vi "update_MagFieldTable_File.vi"(8 "error in (no error)":errorcluster, 11 "MFTObj in":refnum<class "MagFieldTable.lvclass">) -> (0 "error out":errorcluster, 3 "MFTObj out":refnum<class "MagFieldTable.lvclass">)   [LabVIEW 2018]
doc: "updates the MagFieldTables.ini with the most recent data of this MagFieldTable"
uses:
  Classes/MagFieldTable/MagFieldTable.lvclass
  global variables.vi
  <vilib>/Utility/config.llb/Write Key (Double).vi
  Classes/StatusLog/StatusLog.lvclass
  <vilib>/Utility/config.llb/NI_LVConfig.lvlib
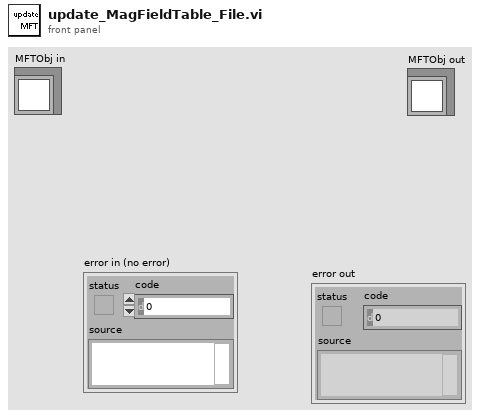
[diagram p1: front panel]
types:
  T1 = typedef "NI_LVConfig.lvlib/Config Data RefNum.ctl" = refnum<k1>
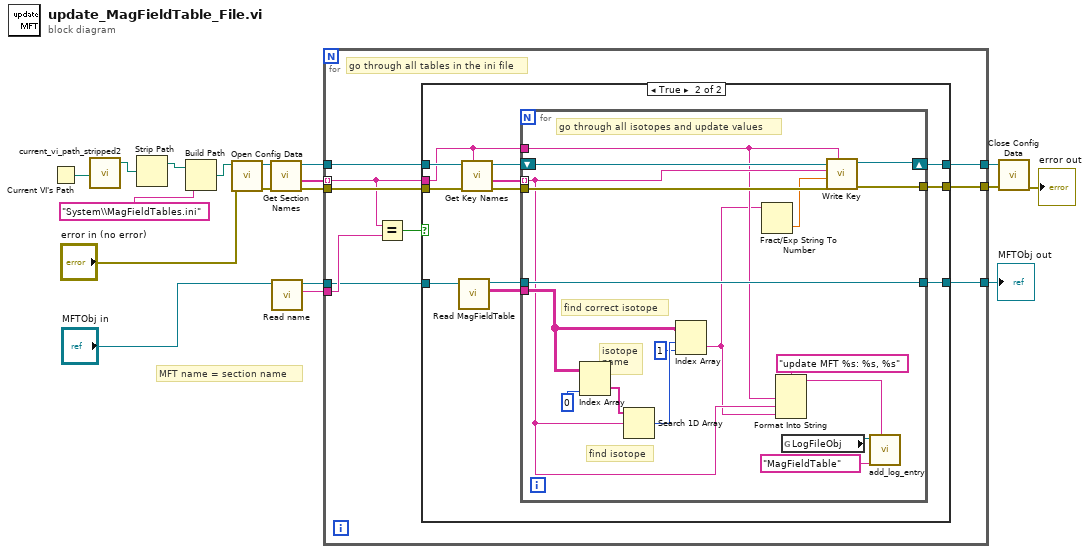
[diagram p0: block diagram]
diagram:
  # "MFT name = section name"
  n1 = Current VI's Path() -> (path=w8:path)
  n2 = call "current_vi_path_stripped2.vi"("current VI Path"=w8) -> ("current VI Path stripped out"=w10:path)  [unwired: 3 in, 1 out]
  n3 = Strip Path(path=w10) -> (stripped path=w9:path)  [unwired: 1 out]
  n4 = Build Path(base path=w9, name or relative path="System\\MagFieldTables.ini") -> (appended path=w7:path)
  n5 = call <vilib>:"Open Config Data.vi"("error in (no error)"="error in (no error)", "configuration file path"=w7) -> ("error out"=w6:errorcluster, "refnum"=w5:T1)  [unwired: 7 in, 1 out]
  n6 = call <vilib>:"Get Section Names.vi"("error in (no error)"=w6, "refnum"=w5) -> ("error out"=w13:errorcluster, "section names"=w14:string[], "refnum out"=w12:T1)  [unwired: 7 in]
  n7 = call-dynamic "Read name.vi"("MagFieldTable in"="MFTObj in") -> ("name"=w16:string, "MagFieldTable out"=w15:refnum<class "MagFieldTable.lvclass">)  [unwired: 8 in, 1 out]
  n8 = for {
    tunnel: w14 -> [w23] mode=indexing
    tunnel: w12 -> [w25]
    tunnel: w13 -> [w24]
    tunnel: w15 -> [w22]
    tunnel: w16 -> [w27]
    tunnel: [w21] -> w18
    tunnel: [w20] -> w17
    tunnel: [w19] -> w3
    # "go through all tables in the ini file"
    n9 = Equal?(x=w23, y=w27) -> (x = y?=w26:bool)
    n10 = case shown="True" w26 {
      tunnel: w25 -> [w30 w42]
      tunnel: w24 -> [w29 w41]
      tunnel: w23 -> [_ w35]
      tunnel: w22 -> [w28 w40]
      tunnel: [w30 w34] -> w21
      tunnel: [w29 w33] -> w20
      tunnel: [w28 w31] -> w19
      frame False {
        # "not the correct MFT"
      }
      frame True {
        n11 = call-dynamic "Read MagFieldTable.vi"("MagFieldTable in"=w40) -> ("MagFieldTable"=w38:string[][], "MagFieldTable out"=w32:refnum<class "MagFieldTable.lvclass">)  [unwired: 8 in, 1 out]
        n12 = call <vilib>:"Get Key Names.vi"("section"=w35, "error in (no error)"=w41, "refnum"=w42) -> ("error out"=w36:errorcluster, "key names"=w39:string[], "refnum out"=w37:T1)  [unwired: 5 in, 1 out]
        n13 = for {
          tunnel: w39 -> [w46] mode=indexing
          tunnel: w38 -> [w58]
          tunnel: w36 -> [w54]
          shift-right: [w53] -> w34
          shift-left: w37 -> [w55]
          tunnel: w35 -> [w45]
          tunnel: [w52] -> w33
          tunnel: w32 -> [w47]
          tunnel: [w47] -> w31
          # "find correct isotope"
          # "go through all isotopes and update values"
          # "isotope\nname"
          # "find isotope"
          n14 = Index Array(array=w58, index (col)=0 ("disabled index (col)")) -> (element=w59:string[])  [unwired: 1 in]
          n15 = Search 1D Array(1D array=w59, element=w46) -> (index of element=w57:i32)  [unwired: 1 in]
          n16 = Index Array(array=w58, index (row)=w57, index (col)=1 ("disabled index (col)")) -> (element=w44:string)
          n17 = Fract/Exp String To Number(string=w44) -> (number=w43:dbl)  [unwired: 3 in, 1 out]
          n18 = Format Into String(format string="update MFT %s: %s, %s", w45, w46, w44) -> (resulting string=w48:string)  [unwired: 2 in, 1 out]
          n19 = global read "global variables.vi" "LogFileObj"() -> (w51:refnum<class "StatusLog.lvclass">)
          n20 = call-poly <vilib>:"Write Key.vi"("section"=w45, "error in (no error)"=w54, "value"=w43, "key"=w46, "refnum"=w55) -> ("error out"=w52:errorcluster, "refnum out"=w53:T1)  [unwired: 4 in, 1 out]
          n21 = call-dynamic "add_log_entry.vi"("new entry"=w48, "log identifiers"="MagFieldTable", "StatusLog in"=w51) -> ()  [unwired: 5 in, 2 out]
        }
      }
    }
  }
  "MFTObj out" <- w3
  n22 = call <vilib>:"Close Config Data.vi"("error in (no error)"=w17, "refnum"=w18) -> ("error out"=→"error out":errorcluster)  [unwired: 8 in, 1 out]
